vi "Peaks_BM_envelope_MaxPeak.vi"(0 "imput sequence":dbl[](array[numeric])=array[10000 elements], 1 "fixed threshold":bool=TRUE, 2 "thres_fix":dbl=4.0, 5 "Noise Level":dbl=2.0, 6 "welche LS ?":u8=3, 7 "RMS miutiplication factor":dbl=2.0, 9 "width 1":i32=4 min=3, 11 "Length of Lsimp":i32=600, 12 "MaximalePeakThreshold":bool=TRUE, 13 "MaxPeak miltiplication factor":dbl=50.0, 14 "Grenz Ampulitude":dbl=10.0) -> (4 "IR with theshold":dbl[][](graph), 10 "FirstPeak":dbl, 15 "Peak Locations":dbl[](array[numeric]))   [LabVIEW 2014]
uses:
  <vilib>/Analysis/5stat.llb/RMS (DBL).vi
  <vilib>/Analysis/NI_AALPro.lvlib
panel:
  out "x ODER y?":bool=TRUE
  out "Locations":dbl[](array[numeric])=[692.7919916615207, 721.1122341831277, 753.8476383495831, 960.8974264145788] caption="Positionen"
  out "Peak Locations":dbl[](array[numeric])=[1292.7973314190772, 1321.1118861367268, 1353.8533784499036, 1560.8995896377965]
  in  "Length of Lsimp 2":i32=600
  in  "width 2":i32=3
  out "Max Peak":dbl=32.66825374816348 format="%.5f"
  out "level echo":dbl=4.0 format="%.2p"
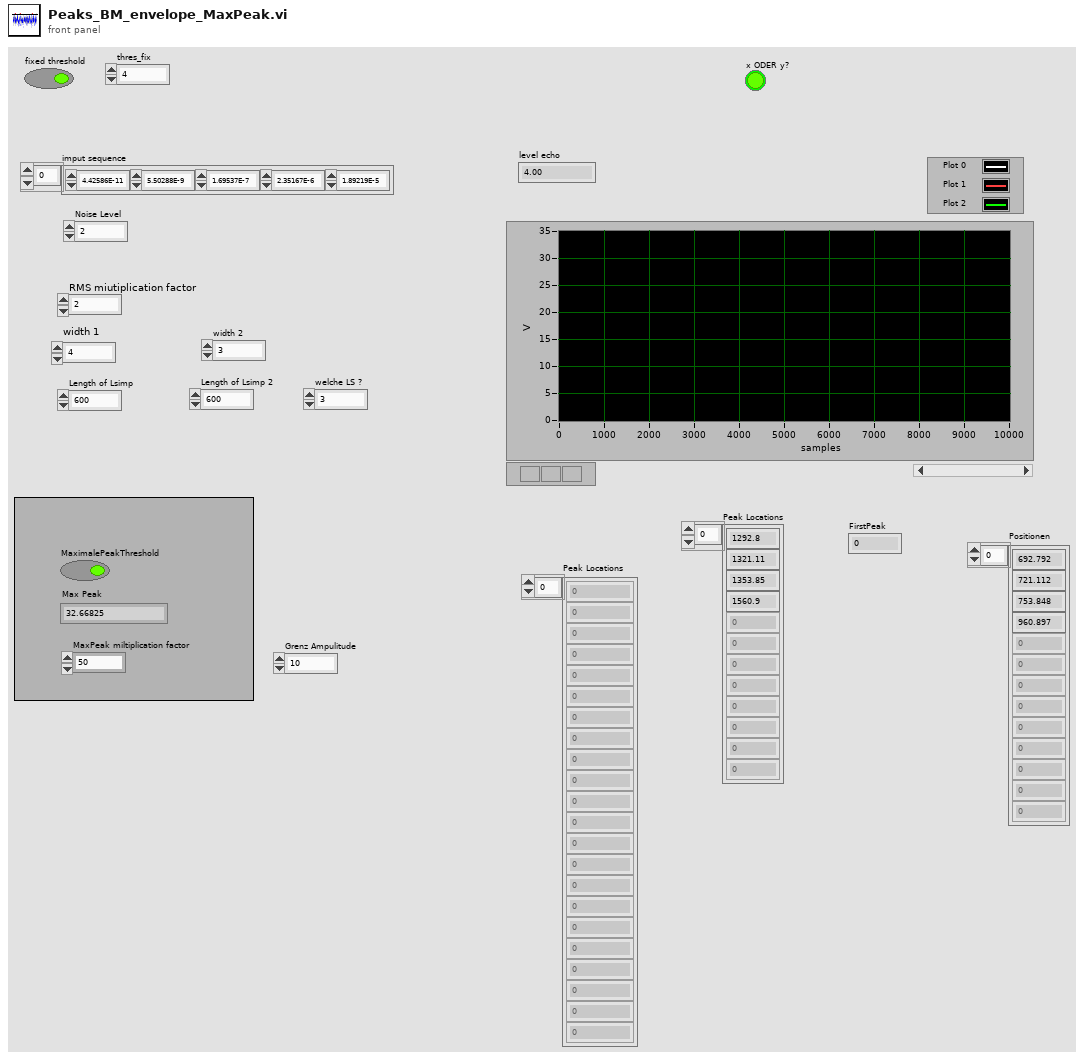
[diagram p1: front panel]
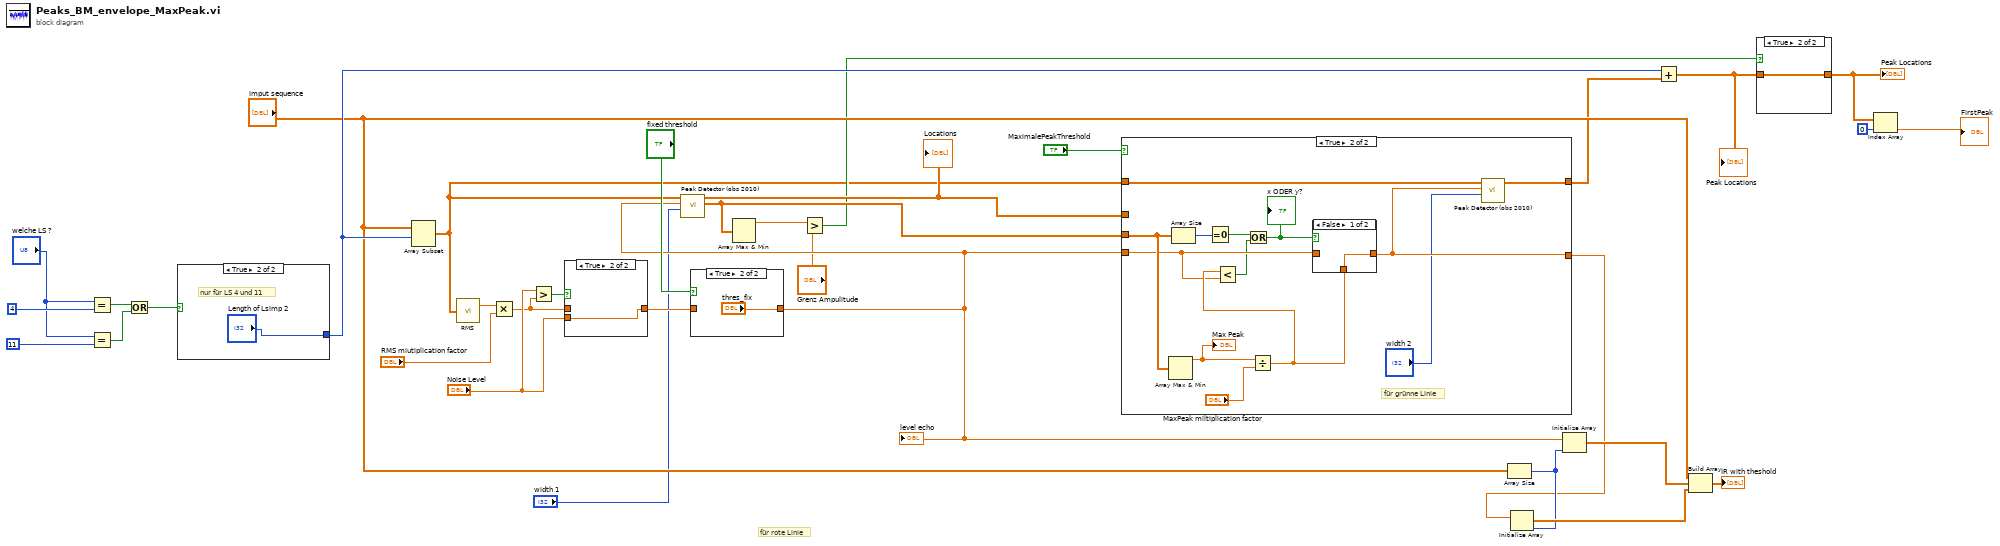
[diagram p0: block diagram]
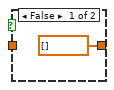
[diagram p2: hidden frame]
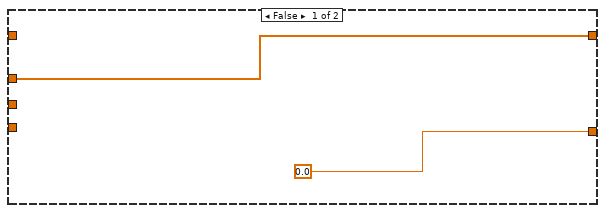
[diagram p3: hidden frame]
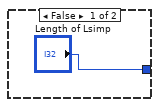
[diagram p5: hidden frame]
diagram:
  # "für rote Linie"
  n1 = Equal?(x="welche LS ?", y=u8 4) -> (x = y?=w3:bool)
  n2 = Equal?(x="welche LS ?", y=u8 11) -> (x = y?=w4:bool)
  n3 = Or(x=w3, y=w4) -> (x .or. y?=w8:bool)
  n4 = case shown="True" w8 {
    tunnel: ["Length of Lsimp" "Length of Lsimp 2"] -> w28
    frame False {
    }
    frame True {
      # "nur für LS 4 und 11"
    }
  }
  n5 = Array Subset(array="imput sequence", index=w28) -> (w2:dbl[])  [unwired: 1 in]
  n6 = call-poly <vilib>:"RMS.vi"("X"=w2) -> ("rms value"=w31:dbl)  [unwired: 1 out]
  n7 = Multiply(x=w31, y="RMS miutiplication factor") -> (x*y=w29:dbl)
  n8 = Greater?(x="Noise Level", y=w29) -> (0:w33:bool)
  n9 = case shown="True" w33 {
    tunnel: w29 -> [w37 _]
    tunnel: "Noise Level" -> [_ w38]
    tunnel: [w37 w38] -> w25
    frame False {
    }
    frame True {
    }
  }
  n10 = case shown="True" "fixed threshold" {
    tunnel: w25 -> [w39 _]
    tunnel: [w39 "thres_fix"] -> w24
    frame False {
    }
    frame True {
    }
  }
  "level echo" <- w24
  n11 = call <vilib>:"Peak Detector (obs 2010).vi"("width"="width 1", "threshold"=w24, "X"=w2) -> ("Amplitudes"=w22:dbl[], "Locations"=w30:dbl[])  [unwired: 4 in, 3 out]
  "Locations" <- w30
  n12 = Array Max & Min(array=w22) -> (max value=w21:dbl)  [unwired: 3 out]
  n13 = Greater?(x=w21, y="Grenz Ampulitude") -> (0:w13:bool)
  n14 = case shown="True" "MaximalePeakThreshold" {
    tunnel: w22 -> [_ w52]
    tunnel: [w42 w44] -> w20
    tunnel: [0.0 w53] -> w16
    tunnel: w30 -> [w42 _]
    tunnel: w24 -> [_ w46]
    tunnel: w2 -> [_ w43]
    frame False {
    }
    frame True {
      # "für grünne Linie"
      n15 = Array Max & Min(array=w52) -> (max value=w51:dbl)  [unwired: 3 out]
      "Max Peak" <- w51
      n16 = Array Size(array=w52) -> (size(s)=w54:i32)
      n17 = Equal To 0?(x=w54) -> (x = 0?=w49:bool)
      n18 = Divide(x=w51, y="MaxPeak miltiplication factor") -> (x/y=w47:dbl)
      n19 = Less?(x=w47, y=w46) -> (x < y?=w45:bool)
      n20 = Or(x=w49, y=w45) -> (x .or. y?=w48:bool)
      "x ODER y?" <- w48
      n21 = case shown="False" w48 {
        tunnel: w46 -> [_ w57]
        tunnel: [w56 w57] -> w53
        tunnel: w47 -> [w56 _]
        frame False {
        }
        frame True {
        }
      }
      n22 = call <vilib>:"Peak Detector (obs 2010).vi"("width"="width 2", "threshold"=w53, "X"=w43) -> ("Locations"=w44:dbl[])  [unwired: 4 in, 4 out]
    }
  }
  n23 = Array Size(array="imput sequence") -> (size(s)=w17:i32)
  n24 = Initialize Array(w16, w17) -> (w18:dbl[])
  n25 = Initialize Array(w24, w17) -> (w19:dbl[])
  n26 = Add(x=w28, y=w20) -> (x+y=w12:dbl[])
  "Peak Locations" <- w12
  n27 = Build Array("imput sequence", w19, w18) -> (→"IR with theshold":dbl[][])
  n28 = case shown="True" w13 {
    tunnel: w12 -> [_ w59]
    tunnel: [dbl[] [] w59] -> w11
    frame False {
    }
    frame True {
    }
  }
  "Peak Locations" <- w11
  n29 = Index Array(array=w11, index=0 ("Index")) -> (element=→"FirstPeak":dbl)
